vi "Read userEventRef.vi"(8 "error in (no error)":errorcluster, 11 "MsgUserEventStopMechanism In":refnum<class "MsgUETaskChannel.lvclass">) -> (0 "error out":errorcluster, 2 "msgUserEvent":refnum<user-event>, 3 "MsgUserEventStopMechanism Out":refnum<class "MsgUETaskChannel.lvclass">)   [LabVIEW 2023, in "TLC_Daemon.lvlib" / "MsgUETaskChannel.lvclass"]
uses:
  MsgUETaskChannel/MsgUETaskChannel.lvclass
  MsgUETaskChannel/MsgUETaskChannel.lvclass/MsgUETaskChannel.ctl
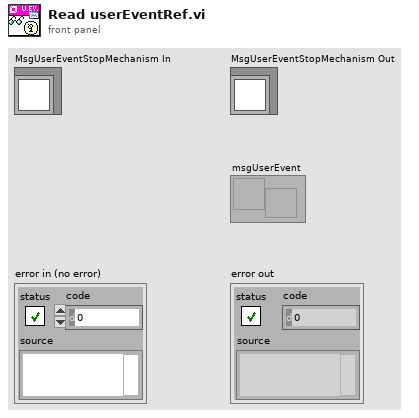
[diagram p1: front panel]
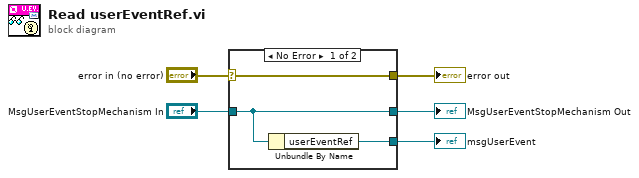
[diagram p0: block diagram]
diagram:
  n1 = case shown="No Error" "error in (no error)" {
    selector: "error in (no error)" -> [w8 w9]
    tunnel: [w8 w9] -> w4
    tunnel: [w7 w10] -> w2
    tunnel: "MsgUserEventStopMechanism In" -> [w7 w10]
    tunnel: [w6 _] -> w1
    frame No Error {
      n2 = Unbundle By Name(w7) -> ("userEventRef"=w6:refnum<user-event>)
    }
    frame Error {
    }
  }
  "error out" <- w4
  "MsgUserEventStopMechanism Out" <- w2
  "msgUserEvent" <- w1
